vi "Building Helper Files DIALOG.vi"(8 "error in (no error)":errorcluster, 11 "Done user event":refnum<user-event>) -> (0 "error out":errorcluster)   [LabVIEW 2023]
panel:
  out "Msg":string
  in  "Close":bool
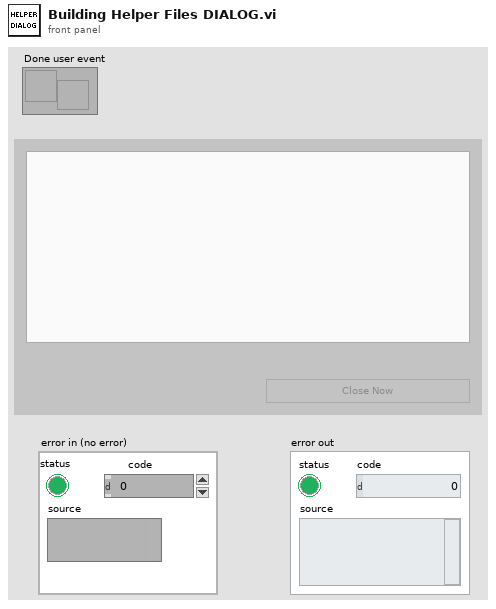
[diagram p1: front panel]
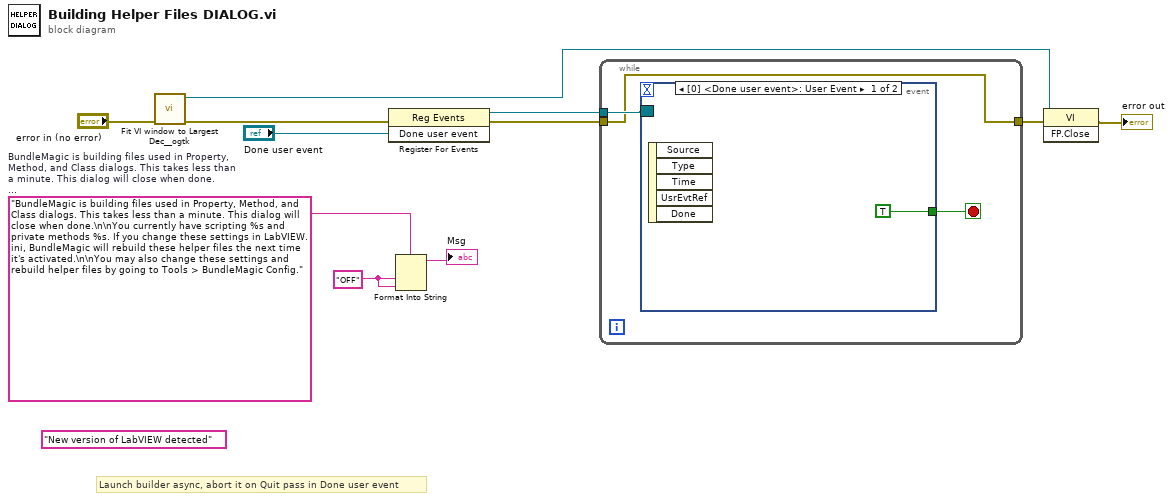
[diagram p0: block diagram]
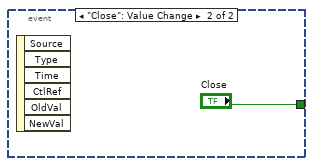
[diagram p2: hidden frame]
diagram:
  (unwired) "New version of LabVIEW detected"
  w7 = "OFF" ("input 1")
  w9 = "BundleMagic is building files used in Property, Method, and Class dialogs. This takes less than a minute. This dialog will close when done.\n\nYou currently have scripting %s and private methods %s. If you change these settings in LabVIEW.ini, BundleMagic will rebuild these helper files the next time it's activated.\n\nYou may also change these settings and rebuild helper files by going to Tools > BundleMagic Config."  # BundleMagic is building files used in Property, Method, and Class dialogs. This takes less than a minute. This dialog will close when done.  You currently have scripting %s and private methods %s. If you change these settings in LabVIEW.ini, BundleMagic will rebuild these helper files the next time it's activated.  You may also change these settings and rebuild helper files by going to Tools > BundleMagic Config.
  # "Launch builder async, abort it on Quit pass in Done user event"
  n1 = call <userlib>:"Fit VI window to Largest Dec__ogtk.vi"("error in (no error)"="error in (no error)") -> ("error out"=w6:errorcluster, "dup VI Ref"=w4:refnum<vi>)  [unwired: 5 in]
  n2 = register-events(error in=w6, "Done user event") -> (reference out=w10:refnum<event-registration>, error out=w2:errorcluster)  [unwired: 1 in]
  n3 = Format Into String(format string=w9, w7, w7) -> (resulting string=→"Msg":string)  [unwired: 2 in, 1 out]
  n4 = while {
    tunnel: w10 -> [w14]
    tunnel: w2 -> [w12]
    tunnel: [w12] -> w1
    stop <- w13 stop-if-true
    n5 = event shown="[0] <Done user event>: User Event" {
      selector: w14 -> [_ _]
      dyn-events: _ -> [_ _]
      timeout: _ -> [_ _]
      tunnel: [TRUE "Close"] -> w13
      event User Event {
        n6 = event-data() -> ()  [unwired: 1 in, 5 out]
      }
      event "Close": Value Change {
        n7 = event-data() -> ()  [unwired: 1 in, 6 out]
      }
    }
  }
  n8 = invoke class="VI" method="FP.Close"(reference=w4, error in=w1) -> (error out=→"error out":errorcluster)  [unwired: 1 in, 2 out]
